vi "Read Call Chain.vi"(11 "TestManagerMsg.Test in":refnum<class "TestManagerMsg.Test.lvclass">) -> (2 "Call Chain":string[](array[string]), 3 "TestManagerMsg.Test out":refnum<class "TestManagerMsg.Test.lvclass">)   [LabVIEW 2013, in "Caraya.lvlib" / "TestManagerMsg.Test.lvclass"]
uses:
  TestManagerMsg.Test.lvclass
  TestManagerMsg.Test.lvclass/TestManagerMsg.Test.ctl
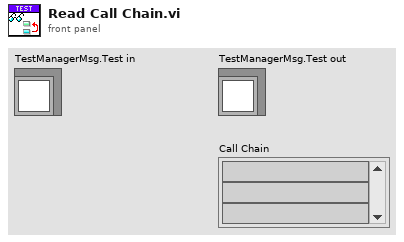
[diagram p1: front panel]
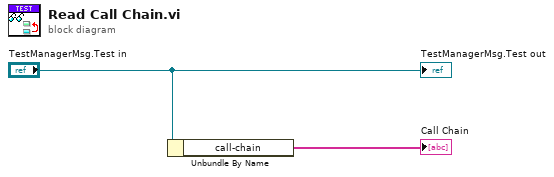
[diagram p0: block diagram]
diagram:
  n1 = Unbundle By Name("TestManagerMsg.Test in") -> ("call-chain"=→"Call Chain":string[])
  "TestManagerMsg.Test out" <- "TestManagerMsg.Test in"
